vi "GlobalVariable.vi"() -> ()   [LabVIEW 2012]
panel:
  out "Vp-pFreq1":cluster{"Vp-p":dbl, "detected frequency":dbl}
  out "Vp-pFreq0":cluster{"Vp-p":dbl, "detected frequency":dbl}
  out "退出采集数据":bool
  out "当前状态":enum16{"等待状态", "采集数据", "退出系统"}(ring)
  in  "采集方式":enum16{"单次有限采样", "多次有限采样", "连续采样"}(ring)
  out "显示点数":dbl
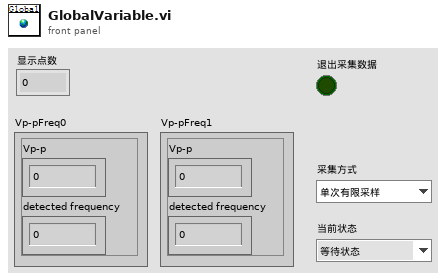
[diagram p1: front panel]
diagram:
